vi "kurtosis.vi"(10 "w":dbl[](array[numeric]), 11 "Input":dbl[][](array[numeric])) -> (3 "kurtosis (K)":dbl)   [LabVIEW 2014]
uses:
  <vilib>/Analysis/baseanly.llb/Vector x A.vi
  <vilib>/Analysis/baseanly.llb/Mean (DBL).vi
  <vilib>/Analysis/NI_AALBase.lvlib
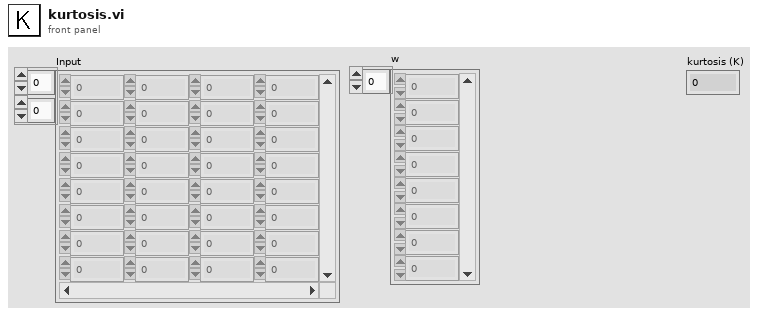
[diagram p1: front panel]
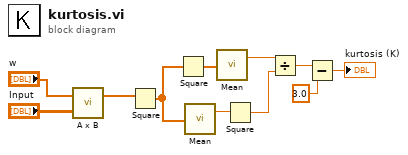
[diagram p0: block diagram]
diagram:
  n1 = call-poly <vilib>:"A x B.vi"("Matrix A"="Input", "Vector V'"="w") -> ("V' x A"=w9:dbl[])  [unwired: 1 out]
  n2 = Square(x=w9) -> (x^2=w7:dbl[])
  n3 = Square(x=w7) -> (x^2=w8:dbl[])
  n4 = call-poly <vilib>:"Mean.vi"("X"=w7) -> ("mean"=w6:dbl)  [unwired: 1 out]
  n5 = call-poly <vilib>:"Mean.vi"("X"=w8) -> ("mean"=w5:dbl)  [unwired: 1 out]
  n6 = Square(x=w6) -> (x^2=w4:dbl)
  n7 = Divide(x=w5, y=w4) -> (x/y=w3:dbl)
  n8 = Subtract(x=w3, y=3.0) -> (x-y=→"kurtosis (K)":dbl)
